vi "Initialize Logging Handler.vi"   [LabVIEW 2022 SP3, in "EDT VIE.lvlib"]
uses:
  EDT VIE.lvlib
  Log Item.ctl
  Log Level.ctl
types:
  T1 = typedef "EDT VIE.lvlib/Log Item.ctl" = cluster{"Log Level":T2, "Message":string}
  T2 = typedef "EDT VIE.lvlib/Log Level.ctl" = enum16{"DEBUG", "INFO", "WARNING", "ERROR", "CRITICAL"}
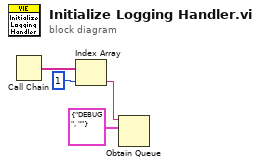
[diagram p0: block diagram]
diagram:
  n1 = Call Chain() -> (call chain=w3:string[])
  n2 = Index Array(array=w3, index=1) -> (element=w1:string)
  n3 = Obtain Queue(name (unnamed)=w1, element data type=T1 {"Log Level"=enum."DEBUG", "Message"=""}) -> ()  [unwired: 3 in, 3 out]
